vi "Asteroid_object.vi"(7 "Asteroid_states":T1, 8 "error in":errorcluster, 11 "DataIn":variant) -> (0 "error out":errorcluster)   [LabVIEW 2017]
uses:
  Asteroid_states.ctl
  Asteroid_data.ctl
  GameConfig/GameConfig_data.ctl
  ManageMovableObjects/HoldData/DataForColision.ctl
  ManageMovableObjects/HoldData/HoldData_mods.ctl
  ManageMovableObjects/ManRef_mods.ctl
  Display/Display_mods.ctl
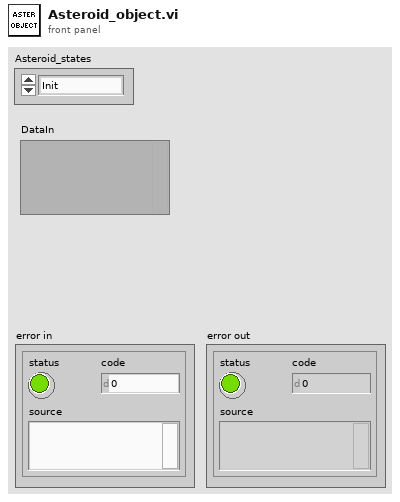
[diagram p1: front panel]
types:
  T1 = typedef "Asteroid_states.ctl" = enum16{"Init", "Move", "Split", "Draw", "Destroy"}
  T2 = typedef "Asteroid_data.ctl" = cluster{"Veloc":dbl, "Direction":dbl, "Size":i32, "displayRef":refnum<vi>, "Max X":dbl, "Max Y":dbl, "Xpos":dbl, "Ypos":dbl, "ID":i32, "Config":T3}
  T3 = typedef "GameConfig_data.ctl" = cluster{"SpaceShip":cluster{"Angle":dbl, "SideLenght":dbl, "MaxLinearVeloc":dbl, "MaxAngularVeloc":dbl, "LinearAceleration":dbl, "AngularAceleration":dbl}, "Physics":cluster{"LinearDragFactor":dbl, "AngularDragFactor":dbl}, "Asteroids":cluster{"MaxSize":dbl, "MaxDivisions":i32, "MaxVeloc":dbl, "MinVeloc":dbl, "Fill":bool}, "Environment":cluster{"MaxAsteroids":i32, "TimeIncrement":dbl, "AsterProbCreation":dbl, "LogEnabled":bool}, "Shots":cluster{"MinTimeShots":dbl, "ShotSize":dbl, "ShotSpeed":dbl}}
  T4 = typedef "HoldData_mods.ctl" = enum16{"Init", "NewAster", "UpdateAster", "RemoveAster", "GetAsterData", "NewShoot", "UpdateShoot", "RemoveShoot", "GetShootData", "End"}
  T5 = typedef "DataForColision.ctl" = cluster{"X":dbl, "Y":dbl, "Size":dbl, "ID":i32}
  T6 = typedef "ManRef_mods.ctl" = enum16{"Init", "NewAster", "MoveAll", "DestroyAster", "NewShoot", "DestroyShot", "CheckColision", "End"}
  T7 = typedef "Display_mods.ctl" = enum16{"Init", "GetBase", "AddAster", "UpdateShip", "AddShoot", "DrawAll", "Clear", "Close"}
  T8 = cluster{"left":i16, "top":i16, "right":i16, "bottom":i16}
  T9 = cluster{"rect":cluster{"left":i16, "top":i16, "right":i16, "bottom":i16}, "Fill":bool}
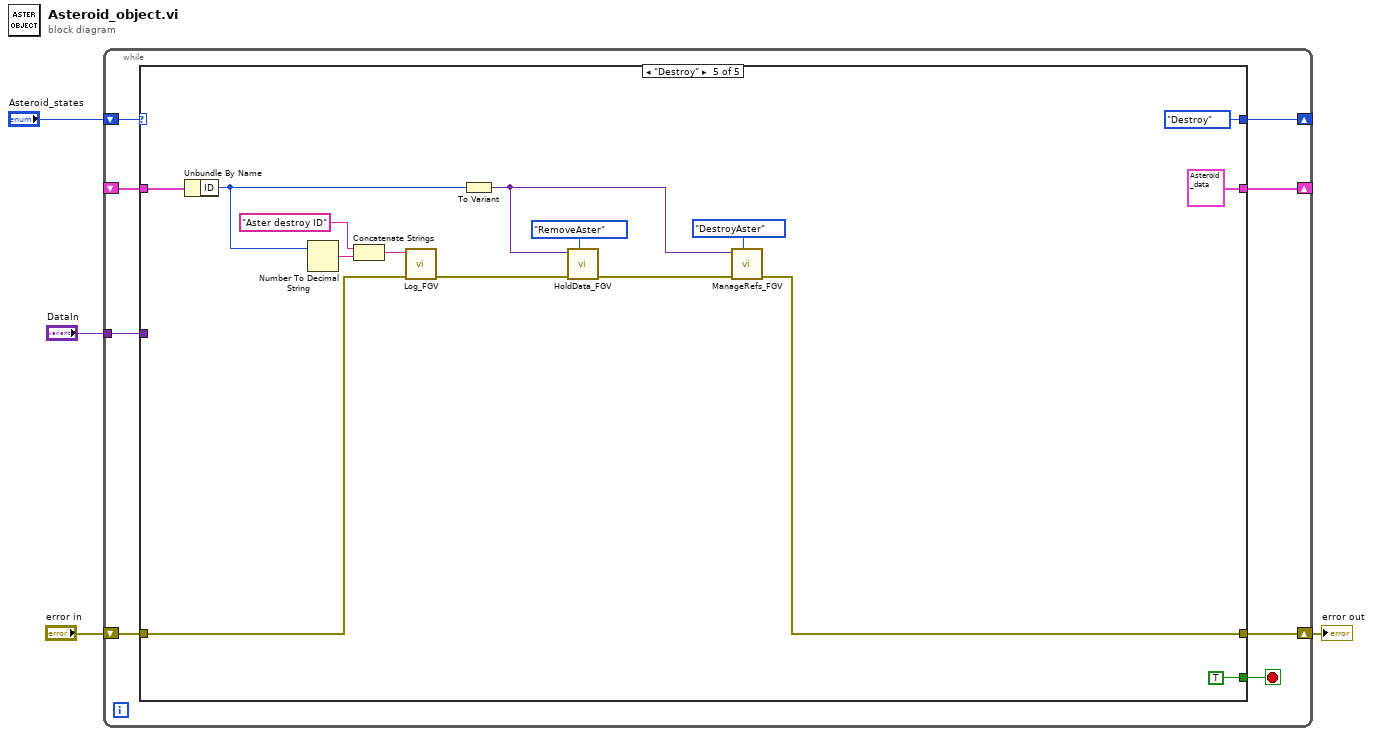
[diagram p0: block diagram]
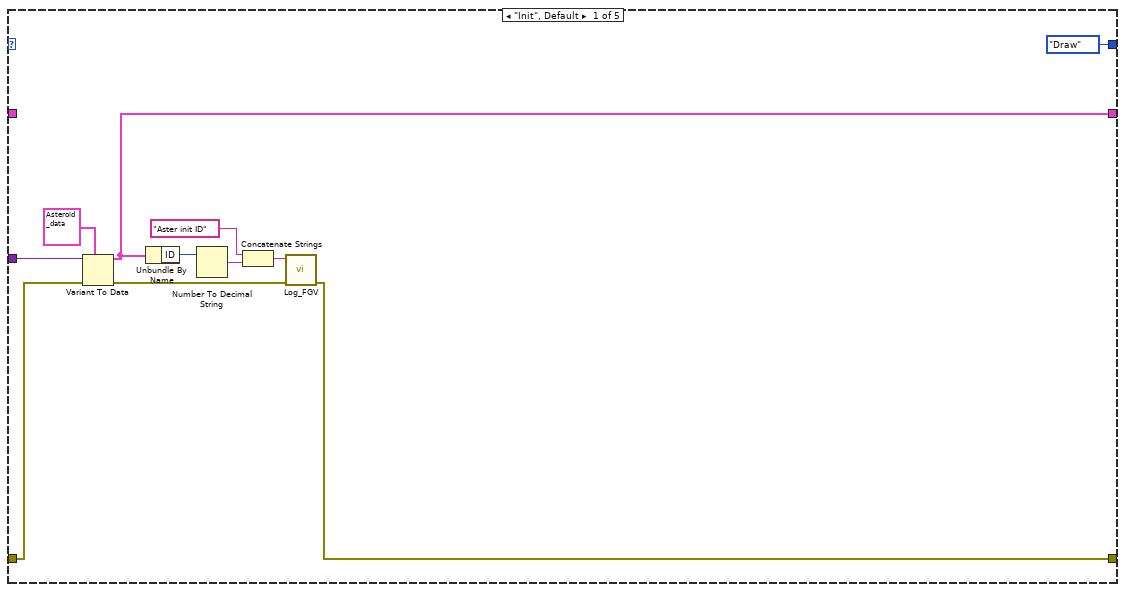
[diagram p2: hidden frame]
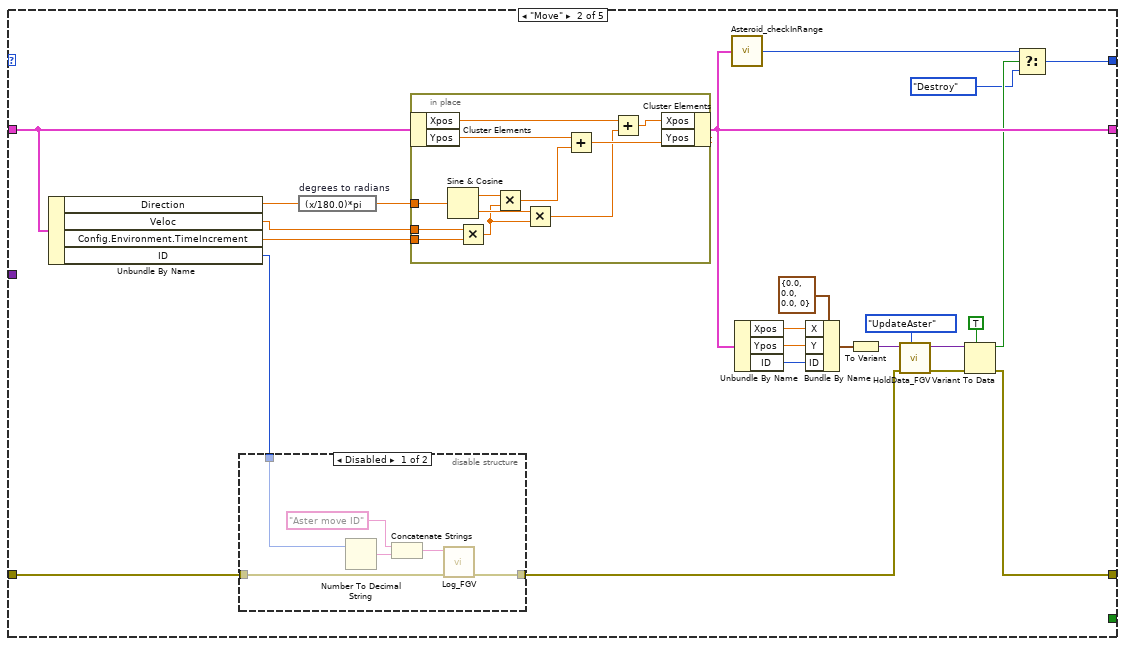
[diagram p3: hidden frame]
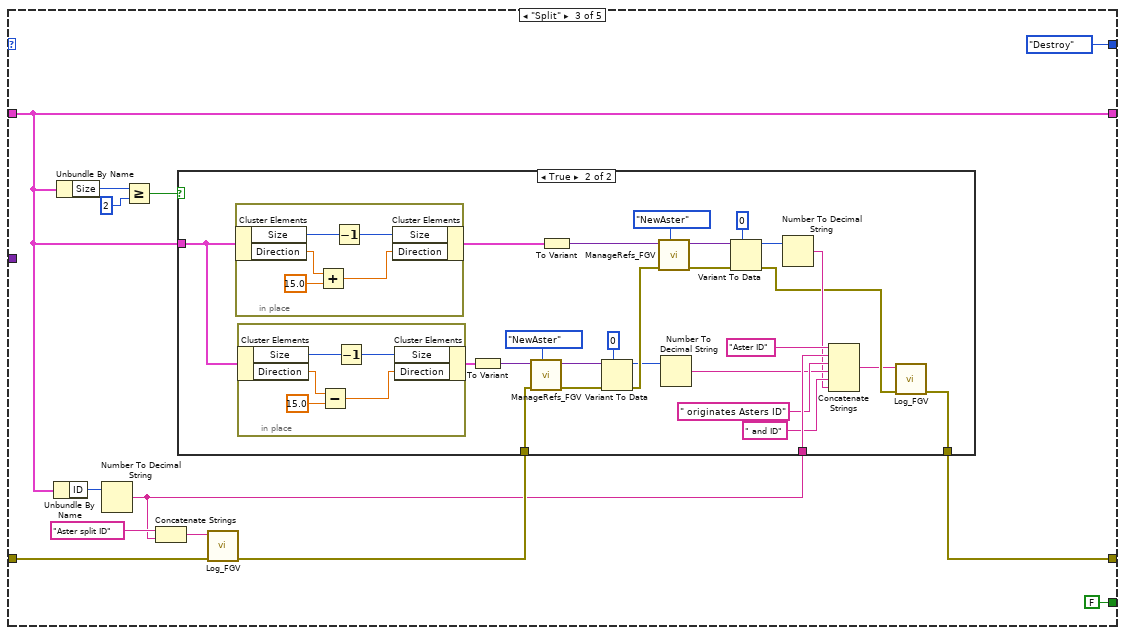
[diagram p5: hidden frame]
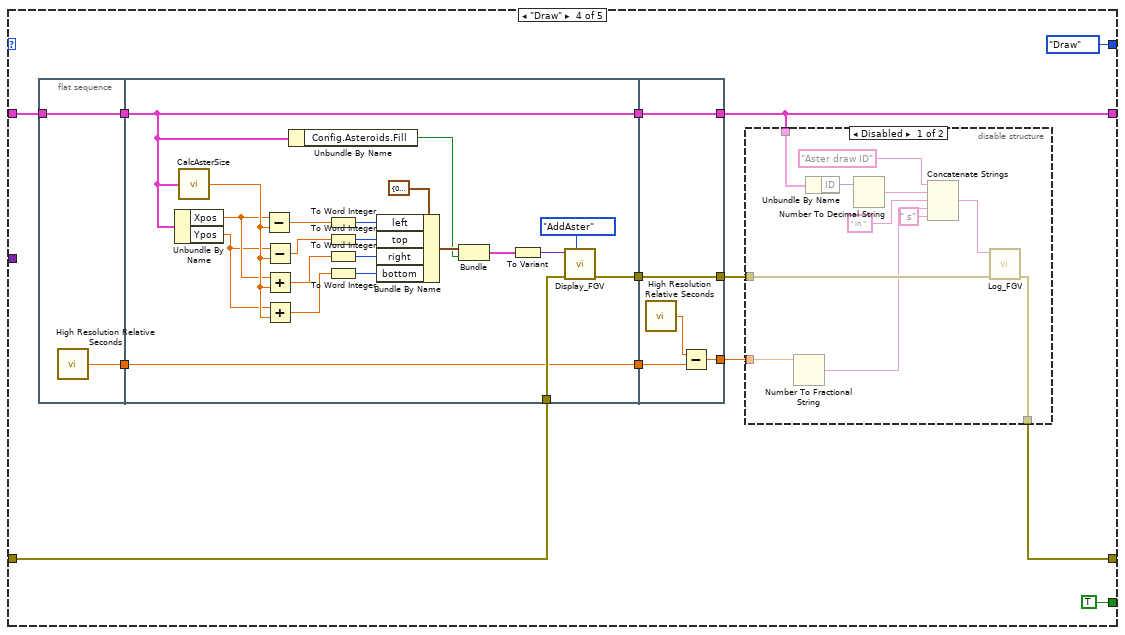
[diagram p7: hidden frame]
diagram:
  n1 = while {
    shift-right: [w10] -> w1
    shift-left: "error in" -> [w11]
    tunnel: "DataIn" -> [w9]
    shift-right: [w8] -> _
    shift-left: _ -> [w7]
    shift-right: [w6] -> _
    shift-left: "Asteroid_states" -> [w12]
    stop <- w5 stop-if-true
    n2 = case shown="\"Destroy\"" w12 {
      tunnel: w11 -> [w14 w41 w70 w127 w176]
      tunnel: [w20 w24 w68 w125 w171] -> w10
      tunnel: w9 -> [w23 _ _ _ _]
      tunnel: [w15 w33 w71 w123 T2 {"Veloc"=0.0, "Direction"=0.0, "Size"=0, "displayRef"=refnum, "Max X"=0.0, "Max Y"=0.0, "Xpos"=0.0, "Ypos"=0.0, "ID"=0, "Config"={"SpaceShip"={"Angle"=30.0, "SideLenght"=2.0, "MaxLinearVeloc"=10.0, "MaxAngularVeloc"=10.0, "LinearAceleration"=1.0, "AngularAceleration"=1.0}, "Physics"={"LinearDragFactor"=1.0, "AngularDragFactor"=1.0}, "Asteroids"={"MaxSize"=6.0, "MaxDivisions"=3, "MaxVeloc"=8.0, "MinVeloc"=1.0, "Fill"=FALSE}, "Environment"={"MaxAsteroids"=10, "TimeIncrement"=0.1, "AsterProbCreation"=0.1, "LogEnabled"=FALSE}, "Shots"={"MinTimeShots"=10.0, "ShotSize"=0.1, "ShotSpeed"=0.1}}} ("AsteroidData")] -> w8
      tunnel: w7 -> [_ w47 w71 w124 w182]
      tunnel: [Asteroid_states."Draw" ("NextState") w30 Asteroid_states."Destroy" ("Asteroid_states") Asteroid_states."Draw" ("NextState") Asteroid_states."Destroy" ("NextState")] -> w6
      tunnel: [_ _ FALSE TRUE TRUE] -> w5
      frame "Init", Default {
        n3 = Variant To Data(error in=w14, type=T2 {"Veloc"=0.0, "Direction"=0.0, "Size"=0, "displayRef"=refnum, "Max X"=0.0, "Max Y"=0.0, "Xpos"=0.0, "Ypos"=0.0, "ID"=0, "Config"={"SpaceShip"={"Angle"=30.0, "SideLenght"=2.0, "MaxLinearVeloc"=10.0, "MaxAngularVeloc"=10.0, "LinearAceleration"=1.0, "AngularAceleration"=1.0}, "Physics"={"LinearDragFactor"=1.0, "AngularDragFactor"=1.0}, "Asteroids"={"MaxSize"=6.0, "MaxDivisions"=3, "MaxVeloc"=8.0, "MinVeloc"=1.0, "Fill"=FALSE}, "Environment"={"MaxAsteroids"=10, "TimeIncrement"=0.1, "AsterProbCreation"=0.1, "LogEnabled"=FALSE}, "Shots"={"MinTimeShots"=10.0, "ShotSize"=0.1, "ShotSpeed"=0.1}}} ("AsteroidData"), Variant=w23) -> (data=w15:T2, error out=w13:errorcluster)
        n4 = Unbundle By Name(w15) -> ("ID"=w19:i32)
        n5 = Number To Decimal String(number=w19) -> (decimal integer string=w18:string)  [unwired: 1 in]
        n6 = Concatenate Strings("Aster init ID" ("Log"), w18) -> (w16:string)
        n7 = call "Log_FGV.vi"("error in"=w13, "Log"=w16) -> ("error out"=w20:errorcluster)  [unwired: 9 in]
      }
      frame "Move" {
        n8 = Unbundle By Name(w47) -> ("Direction"=w44:dbl, "Veloc"=w46:dbl, "Config.Environment.TimeIncrement"=w45:dbl, "ID"=w42:i32)
        n9 = disable-structure shown="Disabled" {
          disable-tunnel: w42 -> [w51 _]
          disable-tunnel: w41 -> [w49 w54]
          disable-tunnel: [w48 w54] -> w32
          frame Disabled {
            n10 = Number To Decimal String(number=w51) -> (decimal integer string=w53:string)  [unwired: 1 in]
            n11 = Concatenate Strings("Aster move ID" ("Log"), w53) -> (w50:string)
            n12 = call "Log_FGV.vi"("error in"=w49, "Log"=w50) -> ("error out"=w48:errorcluster)  [unwired: 9 in]
          }
          frame Enabled {
          }
        }
        n13 = expression code="(x/180.0)*pi" "degrees to radians"(w44) -> (w43:dbl)
        n14 = in-place {
          in-place-border: w46 -> [w66]
          in-place-border: w43 -> [w65]
          in-place-border: w45 -> [w55]
          n15 = in-place-cluster #1(w47) -> ("Xpos"=w57:dbl, "Ypos"=w61:dbl)
          n16 = Sine & Cosine(0:w65) -> (1:w62:dbl, 2:w64:dbl)
          n17 = Multiply(x=w66, y=w55) -> (x*y=w63:dbl)
          n18 = Multiply(x=w62, y=w63) -> (x*y=w60:dbl)
          n19 = Multiply(x=w64, y=w63) -> (x*y=w58:dbl)
          n20 = Add(x=w61, y=w60) -> (x+y=w59:dbl)
          n21 = Add(x=w57, y=w58) -> (x+y=w56:dbl)
          n22 = in-place-cluster #1("Xpos"=w56, "Ypos"=w59) -> (w33:T2)
        }
        n23 = call "Asteroid_checkInRange.vi"("AsteroidData"=w33) -> ("NextState"=w31:T1)
        n24 = Unbundle By Name(w33) -> ("Xpos"=w36:dbl, "Ypos"=w37:dbl, "ID"=w38:i32)
        n25 = Bundle By Name(cluster=T5 {"X"=0.0, "Y"=0.0, "Size"=0.0, "ID"=0} ("DataForColision"), "X"=w36, "Y"=w37, "ID"=w38) -> (w39:T5)
        n26 = To Variant(anything=w39) -> (Variant=w40:variant)
        n27 = call "HoldData_FGV.vi"("HoldData_mods"=HoldData_mods."UpdateAster", "error in"=w32, "DataIn"=w40) -> ("error out"=w29:errorcluster, "DataOut"=w28:variant)  [unwired: 7 in]
        n28 = Variant To Data(error in=w29, type=TRUE, Variant=w28) -> (data=w26:bool, error out=w24:errorcluster)
        n29 = Select(t=w31, s=w26, f=Asteroid_states."Destroy") -> (s? t:f=w30:T1)
      }
      frame "Split" {
        n30 = Unbundle By Name(w71) -> ("ID"=w72:i32)
        n31 = Unbundle By Name(w71) -> ("Size"=w77:i32)
        n32 = Number To Decimal String(number=w72) -> (decimal integer string=w67:string)  [unwired: 1 in]
        n33 = Greater Or Equal?(x=w77, y=2) -> (x >= y?=w75:bool)
        n34 = Concatenate Strings("Aster split ID" ("Log"), w67) -> (w74:string)
        n35 = call "Log_FGV.vi"("error in"=w70, "Log"=w74) -> ("error out"=w69:errorcluster)  [unwired: 9 in]
        n36 = case shown="True" w75 {
          tunnel: w71 -> [_ w106]
          tunnel: w69 -> [w80 w99]
          tunnel: [w80 w81] -> w68
          tunnel: w67 -> [_ w90]
          frame False {
          }
          frame True {
            n37 = in-place {
              n38 = in-place-cluster #2(w106) -> ("Size"=w116:i32, "Direction"=w114:dbl)
              n39 = Add(x=w114, y=15.0) -> (x+y=w112:dbl)
              n40 = Decrement(x=w116) -> (x-1=w115:i32)
              n41 = in-place-cluster #2("Size"=w115, "Direction"=w112) -> (w104:T2)
            }
            n42 = in-place {
              n43 = in-place-cluster #3(w106) -> ("Size"=w111:i32, "Direction"=w109:dbl)
              n44 = Subtract(x=w109, y=15.0) -> (x-y=w107:dbl)
              n45 = Decrement(x=w111) -> (x-1=w110:i32)
              n46 = in-place-cluster #3("Size"=w110, "Direction"=w107) -> (w100:T2)
            }
            n47 = To Variant(anything=w100) -> (Variant=w102:variant)
            n48 = call "ManageRefs_FGV.vi"("ManRef_mods"=ManRef_mods."NewAster", "error in"=w99, "DataIn"=w102) -> ("error out"=w98:errorcluster, "DataOut"=w96:variant)  [unwired: 7 in]
            n49 = To Variant(anything=w104) -> (Variant=w103:variant)
            n50 = Variant To Data(error in=w98, type=0 ("y"), Variant=w96) -> (data=w88:i32, error out=w95:errorcluster)
            n51 = call "ManageRefs_FGV.vi"("ManRef_mods"=ManRef_mods."NewAster", "error in"=w95, "DataIn"=w103) -> ("error out"=w94:errorcluster, "DataOut"=w92:variant)  [unwired: 7 in]
            n52 = Number To Decimal String(number=w88) -> (decimal integer string=w87:string)  [unwired: 1 in]
            n53 = Variant To Data(error in=w94, type=0 ("y"), Variant=w92) -> (data=w85:i32, error out=w83:errorcluster)
            n54 = Number To Decimal String(number=w85) -> (decimal integer string=w84:string)  [unwired: 1 in]
            n55 = Concatenate Strings("Aster ID" ("string"), w90, " originates Asters ID" ("string"), w87, " and ID" ("string"), w84) -> (w82:string)
            n56 = call "Log_FGV.vi"("error in"=w83, "Log"=w82) -> ("error out"=w81:errorcluster)  [unwired: 9 in]
          }
        }
      }
      frame "Draw" {
        n57 = flat-sequence {
          tunnel: w124 -> [w143]
          tunnel: [w143] -> w122
          tunnel: [w142] -> w119
          tunnel: w127 -> [w152]
          tunnel: w122 -> [w146]
          tunnel: [w147] -> w121
          tunnel: [w146] -> w120
          tunnel: w119 -> [w145]
          tunnel: [w145] -> w118
          tunnel: [w168] -> w123
          tunnel: [w169] -> w126
          tunnel: w121 -> [w169]
          tunnel: w120 -> [w168]
          tunnel: w118 -> [w166]
          tunnel: [w165] -> w117
          frame #0 {
            n58 = call <vilib>:"High Resolution Relative Seconds.vi"() -> ("relative seconds"=w142:dbl)
          }
          frame #1 {
            n59 = Unbundle By Name(w146) -> ("Xpos"=w159:dbl, "Ypos"=w158:dbl)
            n60 = call "CalcAsterSize.vi"("AsteroidData"=w146) -> ("AsteroidSize"=w160:dbl)
            n61 = Subtract(x=w159, y=w160) -> (x-y=w163:dbl)
            n62 = Subtract(x=w158, y=w160) -> (x-y=w161:dbl)
            n63 = Add(x=w159, y=w160) -> (x+y=w154:dbl)
            n64 = Add(x=w158, y=w160) -> (x+y=w153:dbl)
            n65 = Unbundle By Name(w146) -> ("Config.Asteroids.Fill"=w150:bool)
            n66 = To Word Integer(number=w163) -> (16bit integer=w162:i16)
            n67 = To Word Integer(number=w161) -> (16bit integer=w157:i16)
            n68 = To Word Integer(number=w154) -> (16bit integer=w156:i16)
            n69 = To Word Integer(number=w153) -> (16bit integer=w155:i16)
            n70 = Bundle By Name(cluster=T8 {"left"=0, "top"=0, "right"=0, "bottom"=0} ("rect"), "left"=w162, "top"=w157, "right"=w156, "bottom"=w155) -> (w151:T8)
            n71 = Bundle("rect"=w151, "Fill"=w150) -> (w149:T9)  [unwired: 1 in]
            n72 = To Variant(anything=w149) -> (Variant=w148:variant)
            n73 = call "Display_FGV.vi"("Display_mods"=Display_mods."AddAster", "error in"=w152, "variant"=w148) -> ("error out"=w147:errorcluster)  [unwired: 7 in, 1 out]
          }
          frame #2 {
            n74 = call <vilib>:"High Resolution Relative Seconds.vi"() -> ("relative seconds"=w167:dbl)
            n75 = Subtract(x=w167, y=w166) -> (x-y=w165:dbl)
          }
        }
        n76 = disable-structure shown="Disabled" {
          disable-tunnel: w126 -> [w136 w141]
          disable-tunnel: [w135 w141] -> w125
          disable-tunnel: w123 -> [w134 _]
          disable-tunnel: w117 -> [w133 _]
          frame Disabled {
            n77 = Number To Fractional String(number=w133) -> (F-format string=w131:string)  [unwired: 3 in]
            n78 = Unbundle By Name(w134) -> ("ID"=w138:i32)
            n79 = Number To Decimal String(number=w138) -> (decimal integer string=w140:string)  [unwired: 1 in]
            n80 = Concatenate Strings("Aster draw ID" ("Log"), w140, " in " ("string"), w131, " s" ("string")) -> (w139:string)
            n81 = call "Log_FGV.vi"("error in"=w136, "Log"=w139) -> ("error out"=w135:errorcluster)  [unwired: 9 in]
          }
          frame Enabled {
          }
        }
      }
      frame "Destroy" {
        n82 = Unbundle By Name(w182) -> ("ID"=w173:i32)
        n83 = Number To Decimal String(number=w173) -> (decimal integer string=w179:string)  [unwired: 1 in]
        n84 = Concatenate Strings("Aster destroy ID" ("Log"), w179) -> (w178:string)
        n85 = call "Log_FGV.vi"("error in"=w176, "Log"=w178) -> ("error out"=w174:errorcluster)  [unwired: 9 in]
        n86 = To Variant(anything=w173) -> (Variant=w170:variant)
        n87 = call "HoldData_FGV.vi"("HoldData_mods"=HoldData_mods."RemoveAster", "error in"=w174, "DataIn"=w170) -> ("error out"=w172:errorcluster)  [unwired: 7 in, 1 out]
        n88 = call "ManageRefs_FGV.vi"("ManRef_mods"=ManRef_mods."DestroyAster", "error in"=w172, "DataIn"=w170) -> ("error out"=w171:errorcluster)  [unwired: 7 in, 1 out]
      }
    }
  }
  "error out" <- w1
